vi "Filter Check.vi"(10 "Cross CSM Data in":T1, 11 "GlobalLogFilter in":refnum<class "LogFilter.lvclass">) -> (0 "Matched? (dup)":bool, 2 "Cross CSM Data out":T1, 3 "GlobalLogFilter.lvclass (dup)":refnum<class "LogFilter.lvclass">)   [LabVIEW 2020, in "Communicable State Machine.lvlib" / "LogFilter.lvclass"]
uses:
  LogFilter.lvclass
  _CSM_GlobalLog_MSG.ctl
  _CSM_Response Source Message.ctl
  _CSM_GlobalLog_MSG_TYPE.ctl
  Communicable State Machine.lvlib
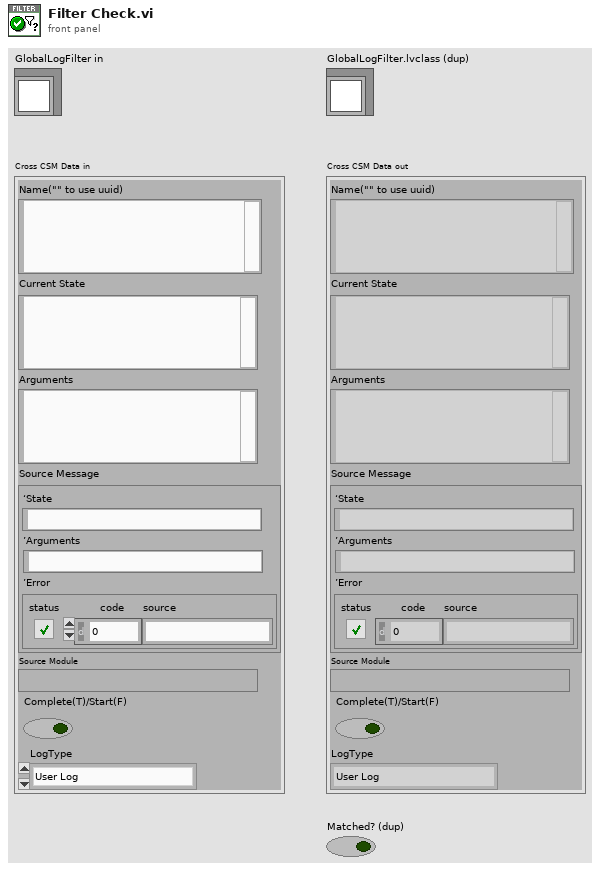
[diagram p1: front panel]
types:
  T1 = typedef "Communicable State Machine.lvlib/_CSM_GlobalLog_MSG.ctl" = cluster{"Name(\"\" to use uuid)":string, "Current State":string, "Arguments":string, "Source Message":T2, "Source Module":string, "Complete(T)/Start(F)":bool, "LogType":T3}
  T2 = typedef "Communicable State Machine.lvlib/_CSM_Response Source Message.ctl" = cluster{"‘State":string, "’Arguments":string, "’Error":errorcluster}
  T3 = typedef "Communicable State Machine.lvlib/_CSM_GlobalLog_MSG_TYPE.ctl" = enum16{"User Log", "State Change", "Status", "Interrupt", "Register", "Unregister", "Error Log", "Module Created", "Module Destroyed"}
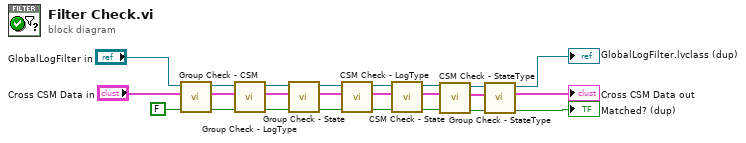
[diagram p0: block diagram]
diagram:
  n1 = call "Group Check - CSM.vi"("Matched Previous?"=FALSE, "Cross CSM Data (in)"="Cross CSM Data in", "GlobalLogFilter.lvclass"="GlobalLogFilter in") -> ("Matched? (dup)"=w18:bool, "Cross CSM Data"=w17:T1, "GlobalLogFilter.lvclass (dup)"=w16:refnum<class "LogFilter.lvclass">)  [unwired: 6 in]
  n2 = call "Group Check - LogType.vi"("Matched Previous?"=w18, "Cross CSM Data (in)"=w17, "GlobalLogFilter.lvclass"=w16) -> ("Matched? (dup)"=w24:bool, "Cross CSM Data"=w20:T1, "GlobalLogFilter.lvclass (dup)"=w23:refnum<class "LogFilter.lvclass">)  [unwired: 6 in]
  n3 = call "Group Check - State.vi"("Matched Previous?"=w24, "Cross CSM Data (in)"=w20, "GlobalLogFilter.lvclass"=w23) -> ("Matched? (dup)"=w12:bool, "Cross CSM Data"=w15:T1, "GlobalLogFilter.lvclass (dup)"=w10:refnum<class "LogFilter.lvclass">)  [unwired: 6 in]
  n4 = call "CSM Check - LogType.vi"("Matched Previous?"=w12, "Cross CSM Data (in)"=w15, "GlobalLogFilter.lvclass"=w10) -> ("Matched? (dup)"=w11:bool, "Cross CSM Data"=w14:T1, "GlobalLogFilter.lvclass (dup)"=w13:refnum<class "LogFilter.lvclass">)  [unwired: 6 in]
  n5 = call "CSM Check - State.vi"("Matched Previous?"=w11, "Cross CSM Data (in)"=w14, "GlobalLogFilter.lvclass"=w13) -> ("Matched? (dup)"=w4:bool, "Cross CSM Data"=w5:T1, "GlobalLogFilter.lvclass (dup)"=w6:refnum<class "LogFilter.lvclass">)  [unwired: 6 in]
  n6 = call "CSM Check - StateType.vi"("Matched Previous?"=w4, "Cross CSM Data (in)"=w5, "GlobalLogFilter.lvclass"=w6) -> ("Matched? (dup)"=w9:bool, "Cross CSM Data"=w8:T1, "GlobalLogFilter.lvclass (dup)"=w7:refnum<class "LogFilter.lvclass">)  [unwired: 6 in]
  n7 = call "Group Check - StateType.vi"("Matched Previous?"=w9, "Cross CSM Data (in)"=w8, "GlobalLogFilter.lvclass"=w7) -> ("Matched? (dup)"=→"Matched? (dup)":bool, "Cross CSM Data"=→"Cross CSM Data out":T1, "GlobalLogFilter.lvclass (dup)"=→"GlobalLogFilter.lvclass (dup)":refnum<class "LogFilter.lvclass">)  [unwired: 6 in]
